vi "INICIA_SERIAL_AUTOGUIDER_QUEUED.vi"(0 "VISA resource name":refnum<visa-resource-name>="COM71", 1 "parity (0:none)":enum16{"None", "Odd", "Even", "Mark", "Space"}(ring), 2 "baud rate (9600)":u32=9600, 3 "stop bits (10: 1 bit)":u16(ring)=10 items=["1.0"=10, "1.5"=15, "2.0"=20], 4 "flow control (0:none)":u16(ring) items=["None", "XON/XOFF", "RTS/CTS", "XON/XOFF & RTS/CTS", "DTR/DSR", "XON/XOFF & DTR/DSR"]) -> (5 "AUTOGUIDER RESOURCE":refnum<visa-resource-name>)   [LabVIEW 2018]
uses:
  Global_Telescopio.vi
  <vilib>/Instr/_visa.llb/VISA Configure Serial Port (Instr).vi
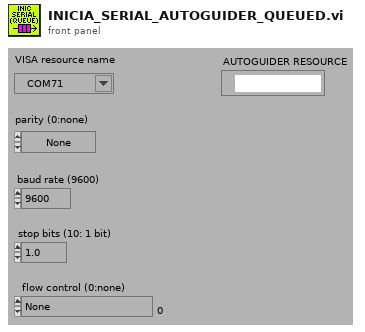
[diagram p1: front panel]
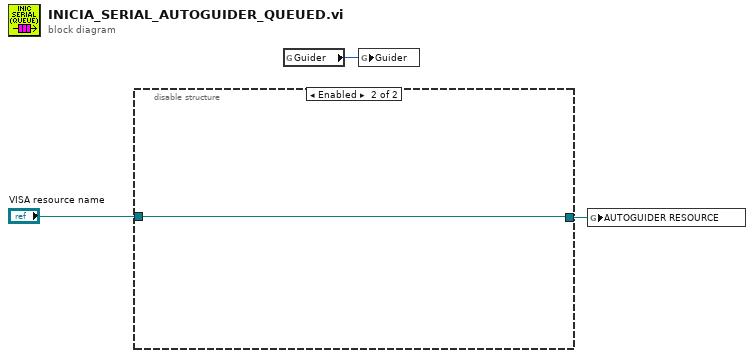
[diagram p0: block diagram]
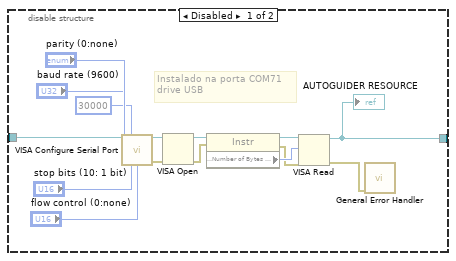
[diagram p2: hidden frame]
diagram:
  n1 = disable-structure shown="Enabled" {
    disable-tunnel: "VISA resource name" -> [w6 w19]
    disable-tunnel: [w4 w19] -> w1
    frame Disabled {
      # "Instalado na porta COM71\ndrive USB"
      n2 = call-poly "VISA Configure Serial Port"("VISA resource name"=w6, "timeout (10sec)"=u32 30000, "baud rate (9600)"="baud rate (9600)", "parity (0:none)"="parity (0:none)", "stop bits (10: 1 bit)"="stop bits (10: 1 bit)", "flow control (0:none)"="flow control (0:none)") -> ("VISA resource name out"=w12:refnum<visa-resource-name>, "error out"=w13:errorcluster)  [unwired: 8 in]
      n3 = VISA Open(error in (no error)=w13, VISA resource name=w12) -> (VISA resource name=w17:refnum<visa-resource-name>, error out=w18:errorcluster)  [unwired: 3 in]
      n4 = property class="Instr"(reference=w17, error in=w18) -> (reference out=w14:refnum<visa-resource-name>, error out=w15:errorcluster, "Serial Settings:Number of Bytes at Serial Port"=w16:u32)
      n5 = VISA Read(VISA resource name=w14, byte count=w16, error in (no error)=w15) -> (VISA resource name out=w4:refnum<visa-resource-name>, error out=w5:errorcluster)  [unwired: 2 out]
      "AUTOGUIDER RESOURCE" <- w4
      n6 = call <vilib>:"General Error Handler.vi"("error in (no error)"=w5) -> ()  [unwired: 10 in, 5 out]
    }
    frame Enabled {
    }
  }
  n7 = global read "Global_Telescopio.vi" "Guider"() -> (w2:i32)
  n8 = global write "Global_Telescopio.vi" "Guider"(w2) -> ()
  n9 = global write "Global_Telescopio.vi" "AUTOGUIDER RESOURCE"(w1) -> ()
